vi "is pool valid.vi"(11 "thread pool in":refnum<class "thread pool.lvclass">) -> (2 "valid":bool, 3 "thread pool out":refnum<class "thread pool.lvclass">)   [LabVIEW 2015, in "thread pool.lvclass"]
uses:
  thread pool.lvclass
  task/strict executor reference.ctl
  thread pool.lvclass/thread pool.ctl
  results reporter/results reporter.lvclass
  task/task.lvclass
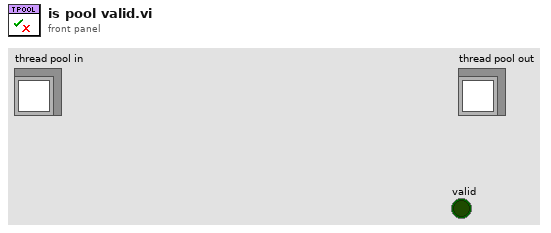
[diagram p1: front panel]
types:
  T1 = typedef "thread pool.lvclass/strict executor reference.ctl" = refnum<vi>
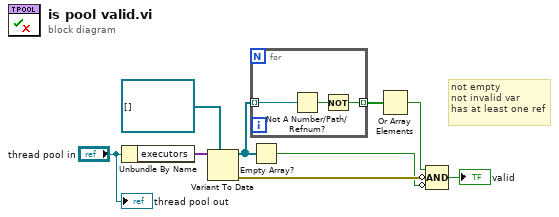
[diagram p0: block diagram]
diagram:
  # "not empty\nnot invalid var\nhas at least one ref"
  n1 = Unbundle By Name("thread pool in") -> ("executors"=w7:variant[])
  n2 = Variant To Data(type=T1[] [], Variant=w7) -> (data=w3:T1[], error out=w4:errorcluster)  [unwired: 1 in]
  n3 = for {
    tunnel: w3 -> [w12] mode=indexing
    tunnel: [w10] -> w6 mode=indexing
    n4 = Not A Number/Path/Refnum?(number/path/refnum=w12) -> (NaN/Path/Refnum?=w11:bool)
    n5 = Not(x=w11) -> (.not. x?=w10:bool)
  }
  n6 = Empty Array?(array=w3) -> (empty?=w2:bool)
  n7 = Or Array Elements(Boolean array=w6) -> (logical OR=w5:bool)
  n8 = Compound Arithmetic op=AND(w5, invert w4, invert w2) -> (→"valid":bool)
  "thread pool out" <- "thread pool in"
